vi "Map String.vi"(0 "default":string, 1 "case matching (sensitive)":T1=enum."system", 4 "key":string, 5 "keys":string[](array[string]), 6 "values":string[](array[string])) -> (2 "index":i32, 3 "valid key":bool, 7 "value":string)   [LabVIEW 2013, in "TLB` Template.lvlib" / "Tools_KeyedArray.lvlib"]
uses:
  Tools_KeyedArray.lvlib
  <vilib>/FTP/util/Case Matching.ctl
  String/Tools_String.lvlib
  <vilib>/FTP/NI_FTP.lvlib
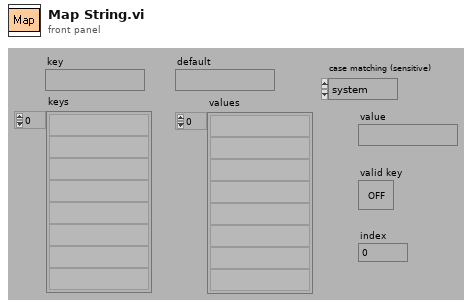
[diagram p1: front panel]
types:
  T1 = typedef "NI_FTP.lvlib/Case Matching.ctl" = enum16{"a != A", "a == A", "system"}
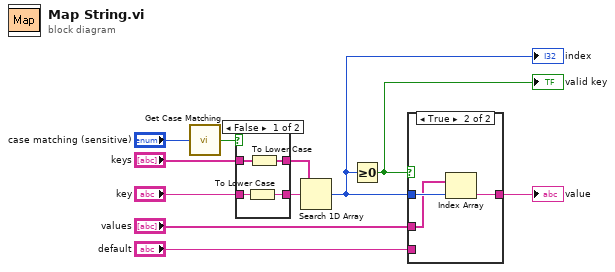
[diagram p0: block diagram]
diagram:
  n1 = call "Get Case Matching.vi"("string matching"="case matching (sensitive)") -> ("match case"=w4:bool)
  n2 = case shown="False" w4 {
    tunnel: "keys" -> [w15 w17]
    tunnel: "key" -> [w13 w16]
    tunnel: [w14 w17] -> w6
    tunnel: [w12 w16] -> w5
    frame False {
      n3 = To Lower Case(string=w13) -> (all lower case string=w12:string)
      n4 = To Lower Case(string=w15) -> (all lower case string=w14:string[])
    }
    frame True {
    }
  }
  n5 = Search 1D Array(1D array=w6, element=w5) -> (index of element=w11:i32)  [unwired: 1 out]
  "index" <- w11
  n6 = Greater Or Equal To 0?(x=w11) -> (x >= 0?=w9:bool)
  "valid key" <- w9
  n7 = case shown="True" w9 {
    tunnel: [w18 w21] -> w10
    tunnel: w11 -> [_ w20]
    tunnel: "default" -> [w18 _]
    tunnel: "values" -> [_ w19]
    frame False {
    }
    frame True {
      n8 = Index Array(array=w19, index=w20) -> (element=w21:string)
    }
  }
  "value" <- w10
